vi "Data_Create Paths Group.vi"(8 "error in (no error)":errorcluster, 11 "variant":variant) -> (0 "error out":errorcluster, 3 "variant out":variant)   [LabVIEW 2015, in "Exposure Process.lvlib"]
uses:
  Exposure Process.lvlib
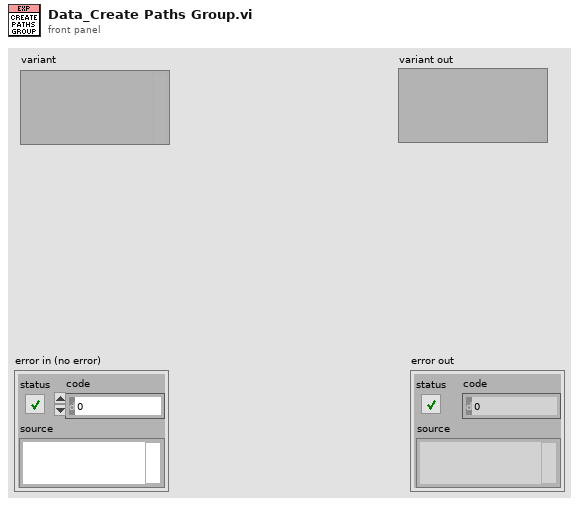
[diagram p1: front panel]
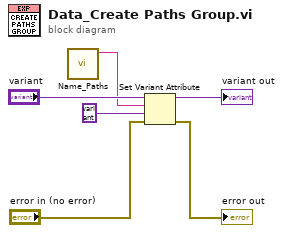
[diagram p0: block diagram]
diagram:
  n1 = call "Name_Paths.vi"() -> ("Name"=w2:string)  [unwired: 11 in]
  n2 = Set Variant Attribute(Variant="variant", name=w2, value=variant, error in="error in (no error)") -> (Variant out=→"variant out":variant, error out=→"error out":errorcluster)  [unwired: 1 out]
